vi "Convert Variant To SGL.vi"(10 "error in (no error)":errorcluster, 11 "Variant":variant) -> (2 "error out":errorcluster, 3 "Numeric":sgl)   [LabVIEW 2020, in "RTAF.lvlib"]
uses:
  RTAF.lvlib
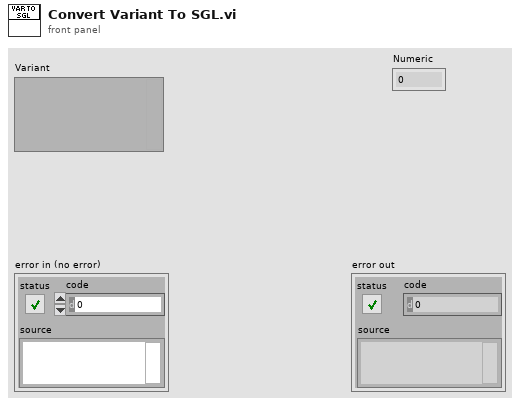
[diagram p1: front panel]
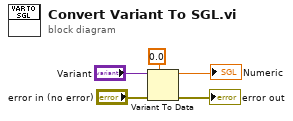
[diagram p0: block diagram]
diagram:
  n1 = Variant To Data(error in="error in (no error)", type=sgl 0.0, Variant="Variant") -> (data=→"Numeric":sgl, error out=→"error out":errorcluster)
